vi "Fermentation_Process (SubVI).vi"(6 "Array in":string[](array[string]), 9 "Temperature Guage":refnum<vi>, 10 "reference in":refnum<vi>, 11 "Boolean in":refnum<vi>) -> (3 "Array out":string[](array[string]))   [LabVIEW 2019]
uses:
  <vilib>/numeric/Random Number (Range) DBL.vi
  ed0096d5-b454-4913-83e5-581dbf1473dc.vi
  f13f5191-991e-4b70-a72b-e0d8466440a7.vi
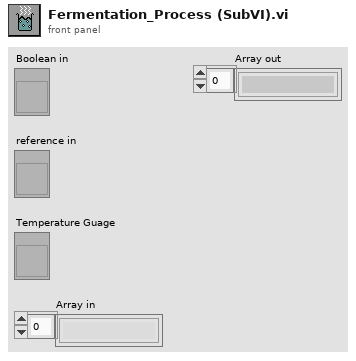
[diagram p1: front panel]
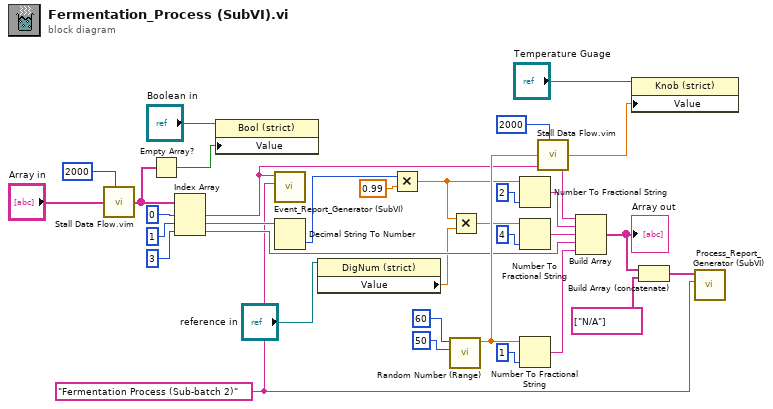
[diagram p0: block diagram]
diagram:
  w4 = "Fermentation Process (Sub-batch 2)" ("Process Name")
  n1 = call "Stall Data Flow.vim"("value in"="Array in", "milliseconds to wait"=u32 2000) -> ("value out"=w12:string[])  [unwired: 1 out]
  n2 = Empty Array?(array=w12) -> (empty?=w11:bool)
  n3 = Index Array(array=w12, index #1=0 ("index"), index #2=1 ("index"), index #3=3 ("index")) -> (element #1=w5:string, element #2=w15:string, element #3=w25:string)
  n4 = property class="Bool (strict)"(reference="Boolean in", "Value"=w11) -> ()  [unwired: 1 in, 2 out]
  n5 = call "Event_Report_Generator (SubVI).vi"("Process Name"=w4, "Booking ID"=w5) -> ()  [unwired: 10 in]
  n6 = Decimal String To Number(string=w15) -> (number=w17:i32)  [unwired: 2 in, 1 out]
  n7 = property class="DigNum (strict)"(reference="reference in") -> ("Value"=w20:dbl)  [unwired: 1 in, 2 out]
  n8 = Multiply(x=w17, y=0.99) -> (x*y=w6:dbl)
  n9 = call-poly <vilib>:"Random Number (Range).vi"("lower bound (0)"=u64 50, "upper bound (100)"=u64 60) -> ("number"=w31:dbl)  [unwired: 9 in]
  n10 = Multiply(x=w6, y=w20) -> (x*y=w22:dbl)
  n11 = Number To Fractional String(number=w6, precision (6)=i16 2) -> (F-format string=w19:string)  [unwired: 2 in]
  n12 = Number To Fractional String(number=w22, precision (6)=i16 4) -> (F-format string=w23:string)  [unwired: 2 in]
  n13 = Number To Fractional String(number=w31, precision (6)=i16 1) -> (F-format string=w28:string)  [unwired: 2 in]
  n14 = call "Stall Data Flow.vim"("value in"=w31, "milliseconds to wait"=u32 2000) -> ("value out"=w32:dbl)  [unwired: 1 out]
  n15 = Build Array(w5, w19, w23, w25, w28) -> (w2:string[])
  "Array out" <- w2
  n16 = property class="Knob (strict)"(reference="Temperature Guage", "Value"=w32) -> ()  [unwired: 1 in, 2 out]
  n17 = Build Array (concatenate)(w2, string[] ["N/A"] ("array")) -> (w3:string[])
  n18 = call "Process_Report_Generator (SubVI).vi"("Process Name"=w4, "Process Information"=w3) -> ()  [unwired: 10 in]
